vi "Rej_szybka_obwiednia.vi"(6 "Liczba probek (200)":i32(slide)=200 min=0 max=400 step=20 scale=0.0..400.0, 7 "#Cores (1)":i32=1, 8 "error in (no error)":errorcluster, 11 "Wfm in":waveform(dbl)) -> (0 "error out":errorcluster, 2 "Wfm min out":waveform(dbl), 3 "Wfm max out":waveform(dbl))   [LabVIEW 2013]
doc: "Liczy obwiednie (gorna -> max i dolna -> min) sygnalu\nLiczba probek zadawana"
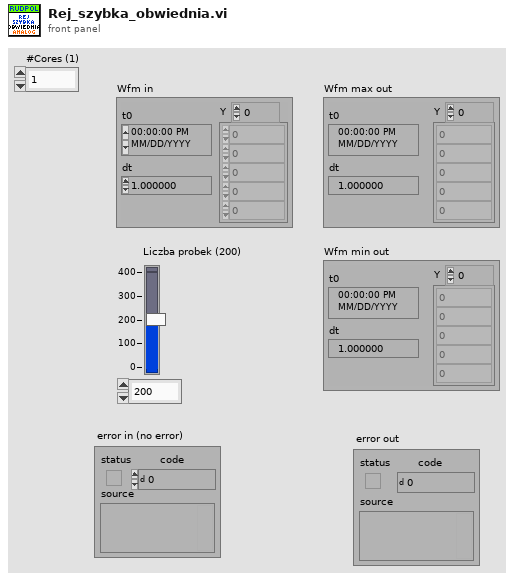
[diagram p1: front panel]
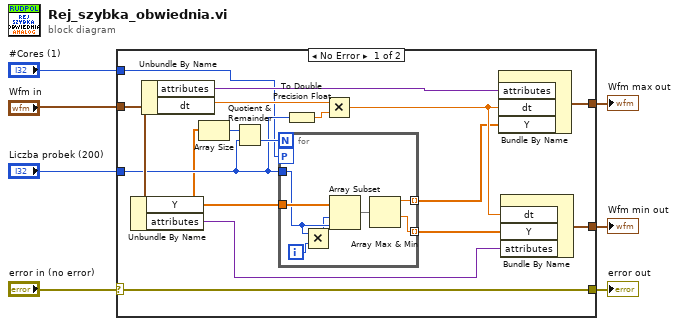
[diagram p0: block diagram]
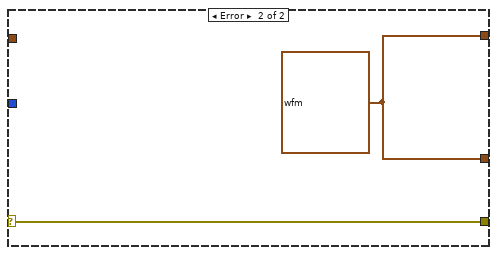
[diagram p2: hidden frame]
diagram:
  n1 = case shown="No Error" "error in (no error)" {
    selector: "error in (no error)" -> [w23 w32]
    tunnel: [w23 w32] -> w7
    tunnel: [w17 w31] -> w5
    tunnel: [w16 w31] -> w4
    tunnel: "Wfm in" -> [w15 _]
    tunnel: "Liczba probek (200)" -> [w14 _]
    tunnel: "#Cores (1)" -> [w10 _]
    frame No Error {
      n2 = Unbundle By Name(w15) -> ("Y"=w11:dbl[], "attributes"=w13:variant)
      n3 = Unbundle By Name(w15) -> ("attributes"=w12:variant, "dt"=w22:dbl)
      n4 = Array Size(array=w11) -> (size(s)=w20:i32)
      n5 = Quotient & Remainder(x=w20, y=w14) -> (floor(x/y)=w19:i32)  [unwired: 1 out]
      n6 = for {
        N: w19 -> [_]
        tunnel: w14 -> [w28]
        tunnel: w11 -> [w30]
        workers-P: w10 -> [_]
        tunnel: [w25] -> w9 mode=indexing
        tunnel: [w24] -> w8 mode=indexing
        i -> [w29]
        n7 = Multiply(x=w28, y=w29) -> (x*y=w27:i32)
        n8 = Array Subset(array=w30, index=w27, length=w28) -> (w26:dbl[])
        n9 = Array Max & Min(array=w26) -> (max value=w24:dbl, min value=w25:dbl)  [unwired: 2 out]
      }
      n10 = To Double Precision Float(number=w14) -> (double precision float=w18:dbl)
      n11 = Multiply(x=w22, y=w18) -> (x*y=w21:dbl)
      n12 = Bundle By Name("attributes"=w12, "dt"=w21, "Y"=w8) -> (w16:waveform(dbl))  [unwired: 1 in]
      n13 = Bundle By Name("dt"=w21, "Y"=w9, "attributes"=w13) -> (w17:waveform(dbl))  [unwired: 1 in]
    }
    frame Error {
      w31 = waveform(dbl) {"t0"=timestamp(0 s since 1904-01-01), "dt"=1.0, "Y"=[]}
    }
  }
  "Wfm max out" <- w4
  "Wfm min out" <- w5
  "error out" <- w7
